vi "IDS_displacement_getAxisDisplacement.vi"(8 "error in (no error)":errorcluster, 10 "axis":i32, 11 "deviceHandle":i32) -> (0 "error out":errorcluster, 2 "displacement":i64, 3 "deviceHandle out":i32)   [LabVIEW 2016]
doc: "int IDS_DLL IDS_displacement_getAxisDisplacement(const int axis, int64_t * displacement);"
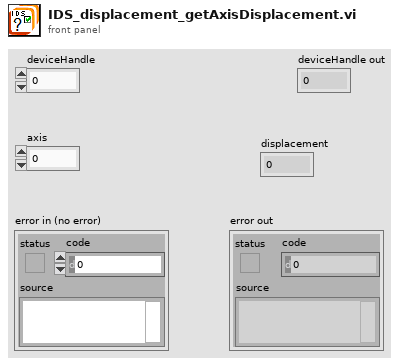
[diagram p1: front panel]
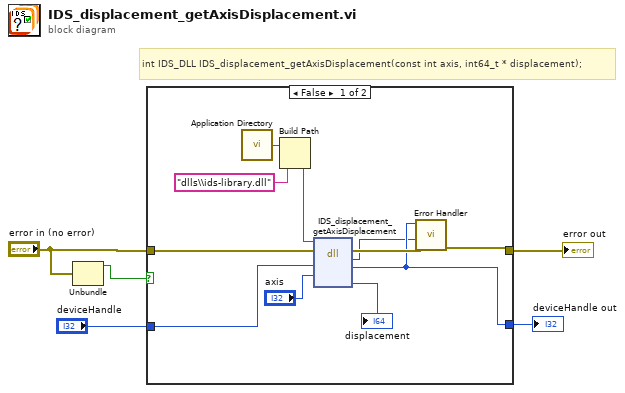
[diagram p0: block diagram]
diagram:
  # "int IDS_DLL IDS_displacement_getAxisDisplacement(const int axis, int64_t * displacement);"
  n1 = Unbundle("error in (no error)") -> ("status"=w1:bool)  [unwired: 2 out]
  n2 = case shown="False" w1 {
    tunnel: "error in (no error)" -> [w15 w18]
    tunnel: [w12 w18] -> w5
    tunnel: "deviceHandle" -> [w11 w17]
    tunnel: [w10 w17] -> w3
    frame False {
      n3 = call <vilib>:"Application Directory.vi"() -> ("Application Directory"=w8:path)
      n4 = Build Path(base path=w8, name or relative path="dlls\\ids-library.dll" ("ipAddress")) -> (appended path=w6:path)
      n5 = dll-call lib="C:/Users/matheus/Desktop/LabVIEW_Draft_V1.6.0/dlls/ids-library.dll" fn="IDS_displacement_getAxisDisplacement"(path in=w6, error in=w15, "deviceHandle"=w11, "axis"="axis") -> (error out=w13:errorcluster, "return type"=w9:i32, "deviceHandle"=w10:i32, "Displacement"=→"displacement":i64)  [unwired: 3 in, 1 out]
      n6 = call "Error Handler.vi"("error in (no error)"=w13, "error code"=w9, "deviceHandle"=w10) -> ("error out"=w12:errorcluster)  [unwired: 7 in, 1 out]
    }
    frame True {
    }
  }
  "error out" <- w5
  "deviceHandle out" <- w3
